vi "ADIS16448_RoboRIO_Teensy_Calibrate.vi"(8 "error in":errorcluster, 11 "SerialPortRef":T1) -> (0 "error out":errorcluster, 3 "SerialPortRefOut":T1)   [LabVIEW 2016, in "ADIS16448-Teensy.lvlib"]
uses:
  ADIS16448-Teensy.lvlib
  <vilib>/Rock Robotics/WPI/SerialPort/WPI_SerialPortRef.ctl
  Util_Functions.ctl
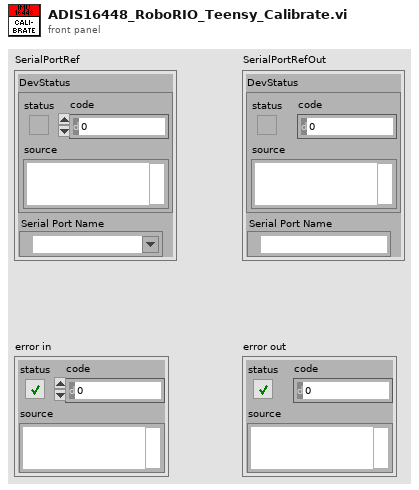
[diagram p1: front panel]
types:
  T1 = typedef "WPI_SerialPortRef.ctl" = cluster{"DevStatus":errorcluster, "Serial Port Name":refnum<visa-resource-name>}
  T2 = typedef "Util_Functions.ctl" = enum16{"None", "Calibrate"}
  T3 = enum16{"set", "get", "set reset", "set function"}
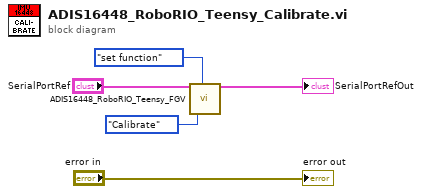
[diagram p0: block diagram]
diagram:
  n1 = call "ADIS16448_RoboRIO_Teensy_FGV.vi"("SerialPortRefIn"="SerialPortRef", "Function"=Util_Functions."Calibrate", "Operation"=T3."set function") -> ("SerialPortRefOut"=→"SerialPortRefOut":T1)  [unwired: 11 in, 5 out]
  "error out" <- "error in"
